vi "circuit sensor.vi"() -> (3 "Property (str)":string=" 0")   [LabVIEW 2019]
uses:
  <vilib>/httpClient/LabVIEWHTTPClient.lvlib
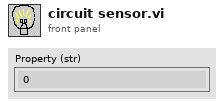
[diagram p1: front panel]
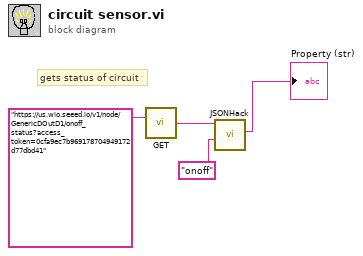
[diagram p0: block diagram]
diagram:
  # "gets status of circuit"
  n1 = call <vilib>:"GET.vi"("url"="https://us.wio.seeed.io/v1/node/GenericDOutD1/onoff_status?access_token=0cfa9ec7b969178704949172d77dbd41") -> ("body"=w3:string)  [unwired: 11 in, 3 out]
  n2 = call "JSONHack.vi"("search name"="onoff", "JSON in"=w3) -> ("Property (str)"=→"Property (str)":string)  [unwired: 6 in, 3 out]
